vi "setCost.vi"(8 "error in (no error)":errorcluster, 10 "cost":dbl, 11 "Beverage in":refnum<class "Beverage.lvclass">) -> (0 "error out":errorcluster, 3 "Beverage out":refnum<class "Beverage.lvclass">)   [LabVIEW 2018, in "Beverage.lvclass"]
uses:
  Beverage.lvclass
  Beverage.lvclass/Beverage.ctl
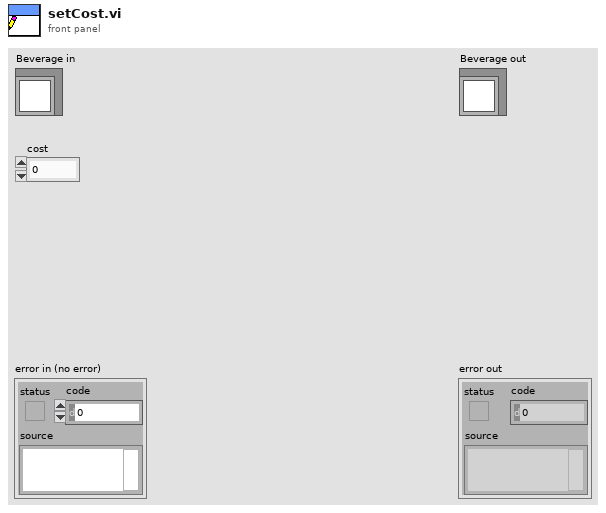
[diagram p1: front panel]
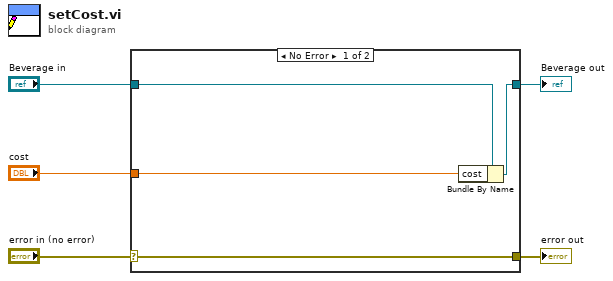
[diagram p0: block diagram]
diagram:
  n1 = case shown="No Error" "error in (no error)" {
    selector: "error in (no error)" -> [w9 w10]
    tunnel: [w9 w10] -> w4
    tunnel: [w7 w11] -> w2
    tunnel: "Beverage in" -> [w8 w11]
    tunnel: "cost" -> [w6 _]
    frame No Error {
      n2 = Bundle By Name(cluster=w8, "cost"=w6) -> (w7:refnum<class "Beverage.lvclass">)
    }
    frame Error {
    }
  }
  "error out" <- w4
  "Beverage out" <- w2
